vi "CAN Cartesian Mecanum.vi"(5 "Scaling Factor":dbl, 8 "Gyro Angle":dbl, 9 "Rotation":dbl, 10 "Y":dbl, 11 "X":dbl) -> ()   [LabVIEW 2012]
uses:
  Robot Global Data.vi
panel:
  in  "error in (no error)":errorcluster
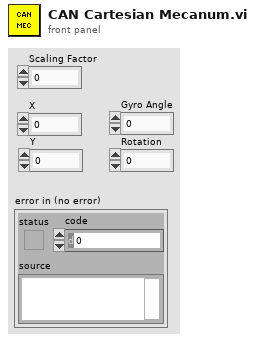
[diagram p1: front panel]
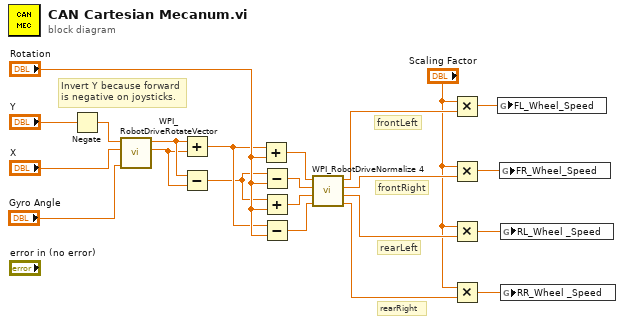
[diagram p0: block diagram]
diagram:
  # "Invert Y because forward is negative on joysticks."
  # "rearLeft"
  # "frontRight"
  # "rearRight"
  # "frontLeft"
  n1 = Negate(x="Y") -> (-x=w6:dbl)
  n2 = call <vilib>:"WPI_RobotDriveRotateVector.vi"("Angle"="Gyro Angle", "X"="X", "Y"=w6) -> ("X'"=w17:dbl, "Y'"=w18:dbl)  [unwired: 7 out]
  n3 = Add(x=w18, y=w17) -> (x+y=w15:dbl)
  n4 = Subtract(x=w18, y=w17) -> (x-y=w13:dbl)
  n5 = Add(x=w15, y="Rotation") -> (x+y=w11:dbl)
  n6 = Subtract(x=w13, y="Rotation") -> (x-y=w12:dbl)
  n7 = Add(x=w13, y="Rotation") -> (x+y=w14:dbl)
  n8 = Subtract(x=w15, y="Rotation") -> (x-y=w16:dbl)
  n9 = call <vilib>:"WPI_RobotDriveNormalize 4.vi"("D"=w16, "C"=w14, "B"=w12, "A"=w11) -> ("D'"=w8:dbl, "C'"=w7:dbl, "B'"=w9:dbl, "A'"=w10:dbl)
  n10 = Multiply(x="Scaling Factor", y=w10) -> (x*y=w5:dbl)
  n11 = Multiply(x="Scaling Factor", y=w9) -> (x*y=w4:dbl)
  n12 = Multiply(x="Scaling Factor", y=w7) -> (x*y=w3:dbl)
  n13 = Multiply(x="Scaling Factor", y=w8) -> (x*y=w2:dbl)
  n14 = global write "Robot Global Data.vi" "FL_Wheel_Speed"(w5) -> ()
  n15 = global write "Robot Global Data.vi" "FR_Wheel_Speed"(w4) -> ()
  n16 = global write "Robot Global Data.vi" "RL_Wheel _Speed"(w3) -> ()
  n17 = global write "Robot Global Data.vi" "RR_Wheel _Speed"(w2) -> ()
